vi "Add Button State.vi"(8 "error in (no error)":errorcluster, 10 "State":refnum<class "BitMap.lvclass">, 11 "Control in":refnum<class "Control.lvclass">) -> (0 "error out":errorcluster, 3 "Control out":refnum<class "Control.lvclass">)   [LabVIEW 2013, in "Control.lvclass"]
doc: "Adds a button state to the array of possible states."
uses:
  Control.lvclass
  <userlib>/BitMan/BitMap class/BitMap.lvclass
  Control.lvclass/Control.ctl
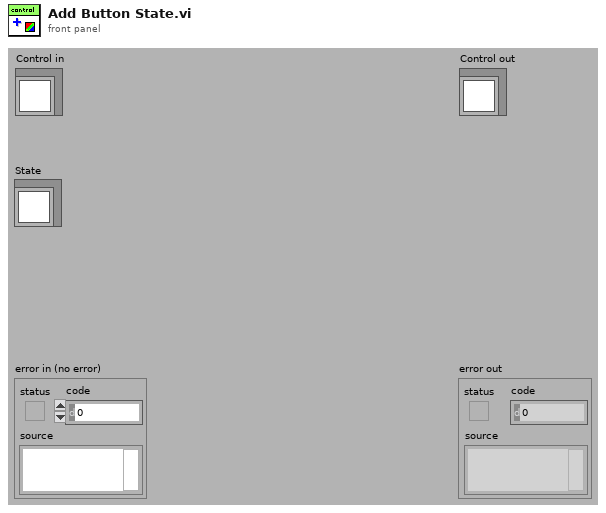
[diagram p1: front panel]
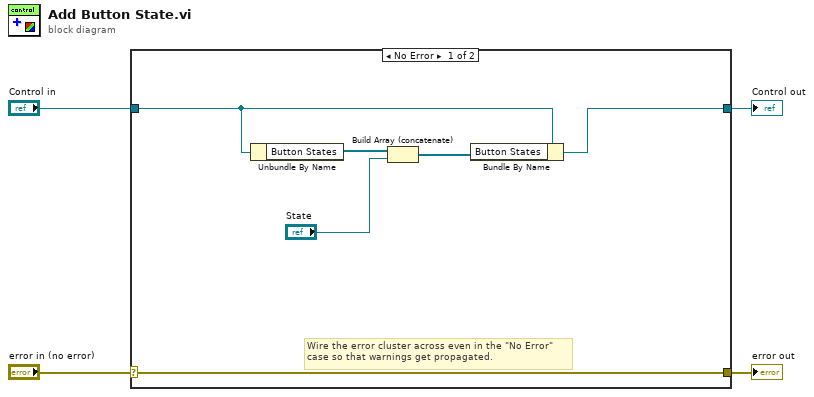
[diagram p0: block diagram]
diagram:
  n1 = case shown="No Error" "error in (no error)" {
    selector: "error in (no error)" -> [w10 w12]
    tunnel: [w10 w12] -> w3
    tunnel: [w8 w11] -> w1
    tunnel: "Control in" -> [w9 w11]
    frame No Error {
      # "Wire the error cluster across even in the \"No Error\"\ncase so that warnings get propagated."
      n2 = Unbundle By Name(w9) -> ("Button States"=w7:refnum<class "BitMap.lvclass">[])
      n3 = Build Array (concatenate)(w7, "State") -> (w6:refnum<class "BitMap.lvclass">[])
      n4 = Bundle By Name(cluster=w9, "Button States"=w6) -> (w8:refnum<class "Control.lvclass">)
    }
    frame Error {
    }
  }
  "error out" <- w3
  "Control out" <- w1
